vi "read_image.vi"(8 "error in (no error)":errorcluster, 11 "Image Path":path) -> (0 "error out":errorcluster, 3 "Output image":T1)   [LabVIEW 2022 SP3]
doc: "Reads image from Image path with extension specified in File type. Accepted file types are jpg, png and bmp."
uses:
  <vilib>/picture/picture.llb/imagedata.ctl
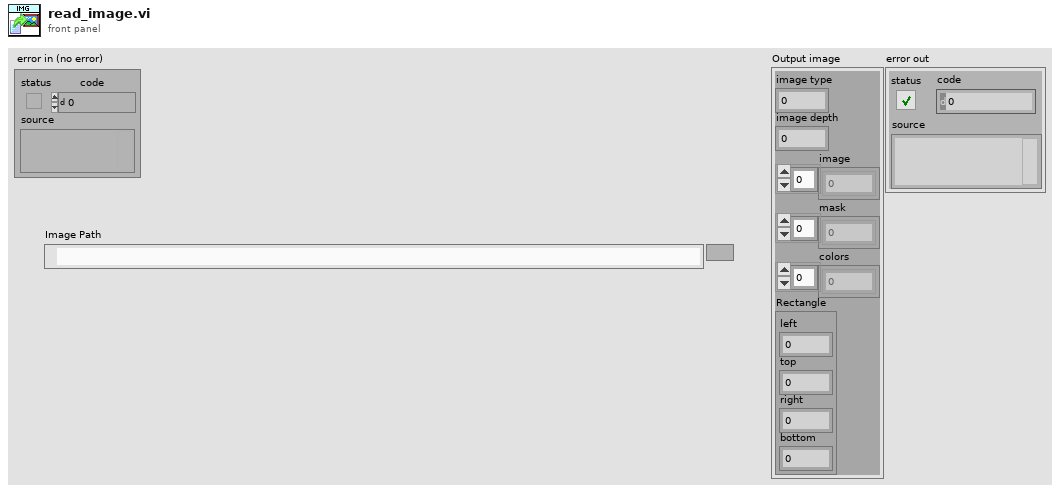
[diagram p1: front panel]
types:
  T1 = typedef "imagedata.ctl" = cluster{"image type":i32, "image depth":i32, "image":u8[], "mask":u8[], "colors":u32[], "Rectangle":cluster{"left":i16, "top":i16, "right":i16, "bottom":i16}}
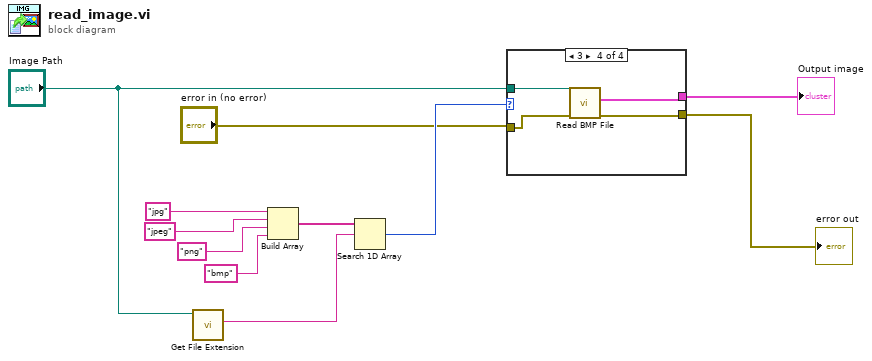
[diagram p0: block diagram]
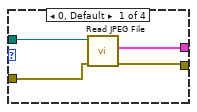
[diagram p2: hidden frame]
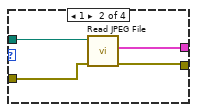
[diagram p3: hidden frame]
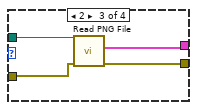
[diagram p4: hidden frame]
diagram:
  n1 = call <vilib>:"Get File Extension.vi"("file"="Image Path") -> ("lowercase file extension"=w6:string)  [unwired: 6 in, 4 out]
  n2 = Build Array("jpg", "jpeg", "png", "bmp") -> (w11:string[])
  n3 = Search 1D Array(1D array=w11, element=w6) -> (index of element=w5:i32)  [unwired: 1 in]
  n4 = case shown="3" w5 {
    tunnel: "Image Path" -> [w15 w19 w23 w27]
    tunnel: [w14 w18 w22 w26] -> w3
    tunnel: "error in (no error)" -> [w13 w16 w21 w25]
    tunnel: [w12 w17 w20 w24] -> w1
    frame 0, Default {
      n5 = call <vilib>:"Read JPEG File.vi"("error in (no error)"=w13, "path to JPEG file"=w15) -> ("error out"=w12:errorcluster, "image data"=w14:T1)  [unwired: 7 in, 1 out]
    }
    frame 1 {
      n6 = call <vilib>:"Read JPEG File.vi"("error in (no error)"=w16, "path to JPEG file"=w19) -> ("error out"=w17:errorcluster, "image data"=w18:T1)  [unwired: 7 in, 1 out]
    }
    frame 2 {
      n7 = call <vilib>:"Read PNG File.vi"("error in (no error)"=w21, "path to PNG file"=w23) -> ("error out"=w20:errorcluster, "image data"=w22:T1)  [unwired: 7 in, 1 out]
    }
    frame 3 {
      n8 = call <vilib>:"Read BMP File.vi"("error in (no error)"=w25, "path to BMP file"=w27) -> ("error out"=w24:errorcluster, "image data"=w26:T1)  [unwired: 7 in, 1 out]
    }
  }
  "Output image" <- w3
  "error out" <- w1
